vi "QuickAverageTwoArrays (SubVI).vi"(1 "B":dbl[](array[numeric]), 2 "A":dbl[](array[numeric])) -> (0 "Average of A and B":dbl[](array[numeric]))   [LabVIEW 2016]
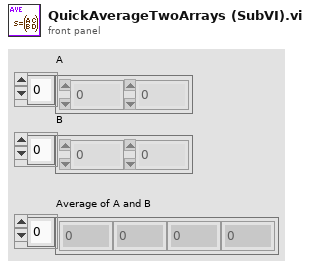
[diagram p1: front panel]
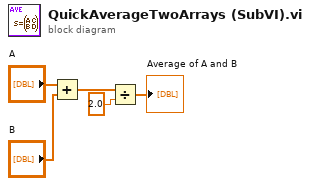
[diagram p0: block diagram]
diagram:
  n1 = Add(x="A", y="B") -> (x+y=w3:dbl[])
  n2 = Divide(x=w3, y=2.0) -> (x/y=→"Average of A and B":dbl[])
